vi "Autonomous Independent.vi"   [LabVIEW 2013]
doc: "This VI is called when autonomous begins, and will automatically be terminated when autonomous ends. You can carry out timed or sensor driven robot movement independently without needing to return to the caller."
uses:
  <vilib>/Rock Robotics/WPI/Solenoid/WPI_SolenoidValue.ctl
  Robot Global Data.vi
  <vilib>/Rock Robotics/WPI/RobotDrive/WPI_RobotDriveGetSetRefNum.vi
  <vilib>/Rock Robotics/WPI/Solenoid/WPI_SolenoidSetEnum.vi
  <vilib>/Rock Robotics/WPI/RobotDrive/WPI_RobotDriveArcadeDrive_Standard(NoSaturation).vi
  <vilib>/Rock Robotics/WPI/Solenoid/Deprecated/WPI_SolenoidGetBool.vi
  <vilib>/Rock Robotics/WPI/Joystick/WPI_JoystickGetSetRefNum.vi
panel:
  # "Be sure to right-click and choose Data Operations>>Make Current Value default if you want to save the array values with the VI"
types:
  T1 = typedef "WPI_JoystickDevRef.ctl" = cluster{"Device":T2}
  T2 = typedef "WPI_JoystickDeviceEnum.ctl" = enum16{"USB 1", "USB 2", "USB 3", "USB 4", "Kinect 1", "Kinect 2"}
  T3 = cluster{"axis 1 (x)":dbl, "axis 2 (y)":dbl, "axis 3 (throttle)":dbl, "axis 4":dbl, "axis 5":dbl, "axis 6":dbl}
  T4 = typedef "WPI_MotorControlDeviceRef.ctl" = cluster{"DeviceStatus":errorcluster, "Type":enum16{"PWM", "CAN"}, "PWM":cluster{"Digital Module":T5, "PWM Channel":T6, "DeadBand":T7}, "CAN":cluster{"Device Number":u8, "Control Mode":T8, "Semaphore":T9, "Max Vout":dbl}, "Invert":bool, "TransformRef":T10, "InvTransformRef":T10}
  T5 = typedef "FPGA_TypedefDigitalModule.ctl" = enum16{"Digital Module 1", "Digital Module 2"}
  T6 = typedef "FPGA_DIOPWMChannel.ctl" = enum8{"PWM 1", "PWM 2", "PWM 3", "PWM 4", "PWM 5", "PWM 6", "PWM 7", "PWM 8", "PWM 9", "PWM 10", "Invalid"}
  T7 = typedef "WPI_PWMDeadband.ctl" = cluster{"Name":string, "maxPositivePwm":i32, "minPositivePwm":i32, "centerPwm":i32, "maxNegativePwm":i32, "minNegativePwm":i32, "angularRange":u16}
  T8 = typedef "WPI_CANJaguar_ControlMode.ctl" = enum8{"Percent VBus", "Current", "Speed", "Position", "Voltage"}
  T9 = typedef "Semaphore RefNum" = refnum<k1>
  T10 = typedef "WPI_PWMTransform_ConPane.ctl" = refnum<vi>
  T11 = typedef "WPI_SolenoidDevRef.ctl" = cluster{"DevStatus":errorcluster, "Solenoid Module":T12, "Forward Solenoid Channel":T13, "Reverse Solenoid Channel":T13}
  T12 = typedef "FPGA_TypedefSolenoidModule.ctl" = enum16{"Solenoid Module 1", "Solenoid Module 2"}
  T13 = typedef "WPI_SolenoidChannel.ctl" = enum8{"Solenoid 1", "Solenoid 2", "Solenoid 3", "Solenoid 4", "Solenoid 5", "Solenoid 6", "Solenoid 7", "Solenoid 8", "Invalid"}
  T14 = typedef "WPI_RobotDriveDevRef.ctl" = cluster{"DevStatus":errorcluster, "Motors[]":T4[], "Square Inputs":bool, "Max Output":dbl, "Isochronous":bool}
  T15 = typedef "WPI_SolenoidValue.ctl" = enum16{"Off", "On", "Forward", "Reverse"}
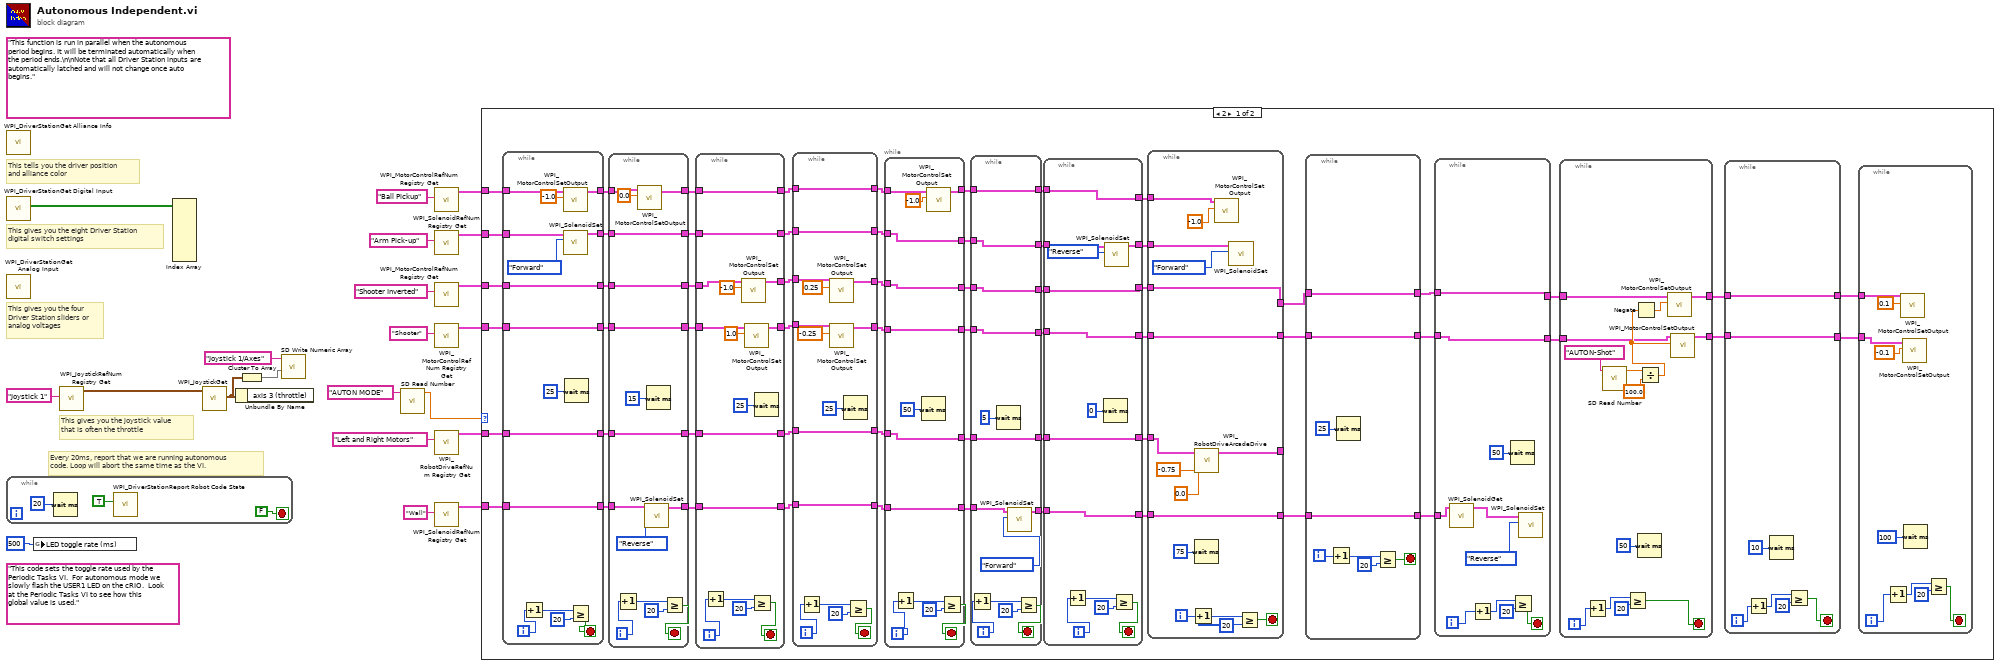
[diagram p0: block diagram]
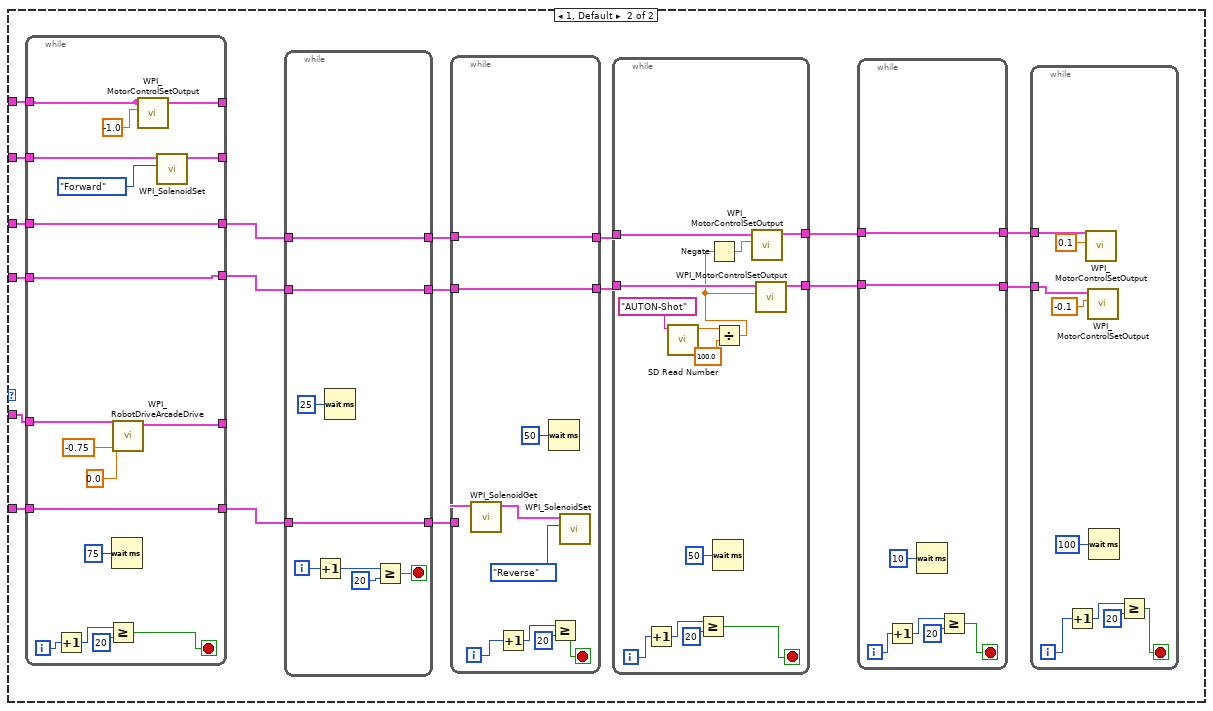
[diagram p2: hidden frame]
diagram:
  (unwired) "This code sets the toggle rate used by the Periodic Tasks VI.  For autonomous mode we slowly flash the USER1 LED on the cRIO.  Look at the Periodic Tasks VI to see how this global value is used."
  (unwired) "This function is run in parallel when the autonomous period begins. It will be terminated automatically when the period ends.\n\nNote that all Driver Station inputs are automatically latched and will not change once auto begins."
  # "Every 20ms, report that we are running autonomous\ncode. Loop will abort the same time as the VI."
  # "This gives you the joystick value\nthat is often the throttle"
  # "This tells you the driver position\nand alliance color"
  # "This gives you the eight Driver Station\ndigital switch settings"
  # "This gives you the four\nDriver Station sliders or\nanalog voltages"
  n1 = call <vilib>:"WPI_DriverStationGet Alliance Info.vi"() -> ()  [unwired: 12 out]
  n2 = call <vilib>:"WPI_DriverStationGet Digital Input.vi"() -> ("Driver Station Digital Input (1-8)"=w21:bool[])  [unwired: 11 out]
  n3 = call <vilib>:"WPI_DriverStationGet Analog Input.vi"() -> ()  [unwired: 12 out]
  n4 = while {
    stop <- FALSE stop-if-true
    n5 = Wait (ms)(milliseconds to wait=u32 20) -> ()  [unwired: 1 out]
    n6 = call <vilib>:"WPI_DriverStationReport Robot Code State.vi"("Autonomous"=TRUE) -> ()  [unwired: 10 in, 1 out]
  }
  n7 = global write "Robot Global Data.vi" "LED toggle rate (ms)"(u32 500 ("LED ms toggle rate")) -> ()
  n8 = call <vilib>:"WPI_JoystickRefNum Registry Get.vi"("refnum name"="Joystick 1") -> ("JoystickDevRef"=w19:T1)  [unwired: 1 in, 9 out]
  n9 = Index Array(array=w21) -> ()  [unwired: 8 in, 8 out]
  n10 = call <vilib>:"WPI_JoystickGet.vi"("JoystickDevRef"=w19) -> ("Axes"=w16:T3)  [unwired: 1 in, 5 out]
  n11 = Unbundle By Name(w16) -> ()  [unwired: 1 out]
  n12 = Cluster To Array(cluster=w16) -> (array=w17:dbl[])
  n13 = call <vilib>:"SD Write Numeric Array.vi"("Numeric Array"=w17, "Name"="Joystick 1/Axes") -> ()  [unwired: 8 in, 2 out]
  n14 = call <vilib>:"SD Read Number.vi"("Name"="AUTON MODE") -> ("Numeric"=w13:dbl)  [unwired: 8 in, 2 out]
  n15 = call <vilib>:"WPI_MotorControlRefNum Registry Get.vi"("refnum name"="Ball Pickup") -> ("MotorControlDevRef"=w1:T4)  [unwired: 9 in, 1 out]
  n16 = call <vilib>:"WPI_SolenoidRefNum Registry Get.vi"("refnum name"="Arm Pick-up") -> ("SolenoidDevRef"=w2:T11)  [unwired: 9 in, 1 out]
  n17 = call <vilib>:"WPI_MotorControlRefNum Registry Get.vi"("refnum name"="Shooter Inverted") -> ("MotorControlDevRef"=w3:T4)  [unwired: 9 in, 1 out]
  n18 = call <vilib>:"WPI_MotorControlRefNum Registry Get.vi"("refnum name"="Shooter") -> ("MotorControlDevRef"=w4:T4)  [unwired: 9 in, 1 out]
  n19 = call <vilib>:"WPI_RobotDriveRefNum Registry Get.vi"("refnum name"="Left and Right Motors") -> ("RobotDriveDevRef"=w6:T14)  [unwired: 9 in, 1 out]
  n20 = call <vilib>:"WPI_SolenoidRefNum Registry Get.vi"("refnum name"="Wall") -> ("SolenoidDevRef"=w5:T11)  [unwired: 9 in, 1 out]
  n21 = case shown="2" w13 {
    tunnel: w6 -> [w76 w265]
    tunnel: w5 -> [w75 w254]
    tunnel: w4 -> [w77 w264]
    tunnel: w3 -> [w78 w263]
    tunnel: w2 -> [w80 w262]
    tunnel: w1 -> [w79 w261]
    frame 2 {
      n22 = while {
        tunnel: w80 -> [w179]
        tunnel: w79 -> [w177]
        tunnel: [w175] -> w71
        tunnel: w78 -> [w175]
        tunnel: w77 -> [w174]
        tunnel: [w174] -> w72
        tunnel: w76 -> [w173]
        tunnel: [w173] -> w73
        tunnel: w75 -> [w172]
        tunnel: [w172] -> w74
        tunnel: [w170] -> w70
        tunnel: [w169] -> w69
        i -> [w180]
        stop <- w181 stop-if-true
        n23 = Increment(x=w180) -> (x+1=w183:i32)
        n24 = call <vilib>:"WPI_MotorControlSetOutput.vi"("Output"=-1.0, "MotorControlDevRef"=w177) -> ("MotorControlDevRef"=w169:T4)  [unwired: 7 in, 2 out]
        n25 = call-poly <vilib>:"WPI_SolenoidSet.vi"("Value"=WPI_SolenoidValue."Forward", "SolenoidDevRef"=w179) -> ("SolenoidDevRef"=w170:T11)  [unwired: 8 in, 1 out]
        n26 = Wait (ms)(milliseconds to wait=u32 25) -> ()  [unwired: 1 out]
        n27 = Greater Or Equal?(x=w183, y=20) -> (x >= y?=w181:bool)
      }
      n28 = while {
        tunnel: w74 -> [w168]
        tunnel: w73 -> [w161]
        tunnel: w72 -> [w160]
        tunnel: w71 -> [w159]
        tunnel: w70 -> [w158]
        tunnel: w69 -> [w156]
        tunnel: [w161] -> w64
        tunnel: [w160] -> w65
        tunnel: [w159] -> w66
        tunnel: [w158] -> w67
        tunnel: [w155] -> w68
        tunnel: [w157] -> w63
        i -> [w163]
        stop <- w164 stop-if-true
        n29 = Increment(x=w163) -> (x+1=w165:i32)
        n30 = call <vilib>:"WPI_MotorControlSetOutput.vi"("Output"=0.0, "MotorControlDevRef"=w156) -> ("MotorControlDevRef"=w155:T4)  [unwired: 7 in, 2 out]
        n31 = call-poly <vilib>:"WPI_SolenoidSet.vi"("Value"=WPI_SolenoidValue."Reverse", "SolenoidDevRef"=w168) -> ("SolenoidDevRef"=w157:T11)  [unwired: 8 in, 1 out]
        n32 = Wait (ms)(milliseconds to wait=u32 15) -> ()  [unwired: 1 out]
        n33 = Greater Or Equal?(x=w165, y=20) -> (x >= y?=w164:bool)
      }
      n34 = while {
        tunnel: w68 -> [w153]
        tunnel: w67 -> [w152]
        tunnel: w66 -> [w150]
        tunnel: w65 -> [w151]
        tunnel: w64 -> [w147]
        tunnel: w63 -> [w146]
        tunnel: [w153] -> w62
        tunnel: [w152] -> w61
        tunnel: [w147] -> w58
        tunnel: [w146] -> w57
        tunnel: [w145] -> w60
        tunnel: [w144] -> w59
        i -> [w140]
        stop <- w141 stop-if-true
        n35 = Increment(x=w140) -> (x+1=w143:i32)
        n36 = call <vilib>:"WPI_MotorControlSetOutput.vi"("Output"=-1.0, "MotorControlDevRef"=w150) -> ("MotorControlDevRef"=w145:T4)  [unwired: 7 in, 2 out]
        n37 = call <vilib>:"WPI_MotorControlSetOutput.vi"("Output"=1.0, "MotorControlDevRef"=w151) -> ("MotorControlDevRef"=w144:T4)  [unwired: 7 in, 2 out]
        n38 = Greater Or Equal?(x=w143, y=20) -> (x >= y?=w141:bool)
        n39 = Wait (ms)(milliseconds to wait=u32 25) -> ()  [unwired: 1 out]
      }
      n40 = while {
        tunnel: w62 -> [w134]
        tunnel: w61 -> [w133]
        tunnel: w60 -> [w137]
        tunnel: w59 -> [w138]
        tunnel: [w134] -> w51
        tunnel: [w133] -> w52
        tunnel: w58 -> [w131]
        tunnel: w57 -> [w132]
        tunnel: [w132] -> w56
        tunnel: [w131] -> w55
        tunnel: [w130] -> w54
        tunnel: [w129] -> w53
        i -> [w125]
        stop <- w126 stop-if-true
        n41 = Increment(x=w125) -> (x+1=w127:i32)
        n42 = call <vilib>:"WPI_MotorControlSetOutput.vi"("Output"=-0.25, "MotorControlDevRef"=w138) -> ("MotorControlDevRef"=w130:T4)  [unwired: 7 in, 2 out]
        n43 = call <vilib>:"WPI_MotorControlSetOutput.vi"("Output"=0.25, "MotorControlDevRef"=w137) -> ("MotorControlDevRef"=w129:T4)  [unwired: 7 in, 2 out]
        n44 = Wait (ms)(milliseconds to wait=u32 25) -> ()  [unwired: 1 out]
        n45 = Greater Or Equal?(x=w127, y=20) -> (x >= y?=w126:bool)
      }
      n46 = while {
        tunnel: w56 -> [w116]
        tunnel: w55 -> [w115]
        tunnel: w54 -> [w114]
        tunnel: w53 -> [w113]
        tunnel: w52 -> [w112]
        tunnel: w51 -> [w123]
        tunnel: [w116] -> w50
        tunnel: [w115] -> w45
        tunnel: [w114] -> w46
        tunnel: [w113] -> w47
        tunnel: [w112] -> w49
        tunnel: [w111] -> w48
        i -> [w118]
        stop <- w119 stop-if-true
        n47 = Increment(x=w118) -> (x+1=w121:i32)
        n48 = Wait (ms)(milliseconds to wait=u32 50) -> ()  [unwired: 1 out]
        n49 = call <vilib>:"WPI_MotorControlSetOutput.vi"("Output"=-1.0, "MotorControlDevRef"=w123) -> ("MotorControlDevRef"=w111:T4)  [unwired: 7 in, 2 out]
        n50 = Greater Or Equal?(x=w121, y=20) -> (x >= y?=w119:bool)
      }
      n51 = while {
        tunnel: w50 -> [w104]
        tunnel: w49 -> [w99]
        tunnel: w48 -> [w98]
        tunnel: w47 -> [w100]
        tunnel: w46 -> [w101]
        tunnel: w45 -> [w102]
        tunnel: [w103] -> w36
        tunnel: [w102] -> w44
        tunnel: [w101] -> w42
        tunnel: [w100] -> w41
        tunnel: [w99] -> w40
        tunnel: [w98] -> w37
        i -> [w107]
        stop <- w106 stop-if-true
        n52 = Increment(x=w107) -> (x+1=w108:i32)
        n53 = Wait (ms)(milliseconds to wait=u32 5) -> ()  [unwired: 1 out]
        n54 = call-poly <vilib>:"WPI_SolenoidSet.vi"("Value"=WPI_SolenoidValue."Forward", "SolenoidDevRef"=w104) -> ("SolenoidDevRef"=w103:T11)  [unwired: 8 in, 1 out]
        n55 = Greater Or Equal?(x=w108, y=20) -> (x >= y?=w106:bool)
      }
      n56 = while {
        tunnel: [w97] -> w43
        tunnel: w44 -> [w97]
        tunnel: w42 -> [w96]
        tunnel: [w96] -> w29
        tunnel: [w95] -> w28
        tunnel: w41 -> [w95]
        tunnel: w40 -> [w88]
        tunnel: [w87] -> w39
        tunnel: [w94] -> w38
        tunnel: w37 -> [w94]
        tunnel: [w93] -> w35
        tunnel: w36 -> [w93]
        i -> [w89]
        stop <- w90 stop-if-true
        n57 = Increment(x=w89) -> (x+1=w92:i32)
        n58 = Wait (ms)(milliseconds to wait=u32 0) -> ()  [unwired: 1 out]
        n59 = call-poly <vilib>:"WPI_SolenoidSet.vi"("Value"=WPI_SolenoidValue."Reverse", "SolenoidDevRef"=w88) -> ("SolenoidDevRef"=w87:T11)  [unwired: 8 in, 1 out]
        n60 = Greater Or Equal?(x=w92, y=20) -> (x >= y?=w90:bool)
      }
      n61 = while {
        tunnel: [w242] -> _
        tunnel: w43 -> [w237]
        tunnel: w39 -> [w236]
        tunnel: w38 -> [w235]
        tunnel: [w234] -> w33
        tunnel: w35 -> [w234]
        tunnel: [w233] -> w30
        tunnel: w29 -> [w233]
        tunnel: w28 -> [w232]
        tunnel: [w232] -> w27
        i -> [w247]
        stop <- w244 stop-if-true
        n62 = Increment(x=w247) -> (x+1=w246:i32)
        n63 = Wait (ms)(milliseconds to wait=u32 75) -> ()  [unwired: 1 out]
        n64 = call-poly <vilib>:"WPI_RobotDriveArcadeDrive.vi"("Y axis value"=-0.75, "X axis value"=0.0, "RobotDriveDevRef"=w237) -> ("RobotDriveDevRef"=w242:T14)  [unwired: 6 in, 2 out]
        n65 = call <vilib>:"WPI_MotorControlSetOutput.vi"("Output"=-1.0, "MotorControlDevRef"=w235) -> ()  [unwired: 7 in, 3 out]
        n66 = call-poly <vilib>:"WPI_SolenoidSet.vi"("Value"=WPI_SolenoidValue."Forward", "SolenoidDevRef"=w236) -> ()  [unwired: 8 in, 2 out]
        n67 = Greater Or Equal?(x=w246, y=20) -> (x >= y?=w244:bool)
      }
      n68 = while {
        tunnel: [w186] -> w34
        tunnel: w33 -> [w186]
        tunnel: [w185] -> w31
        tunnel: w30 -> [w185]
        tunnel: w27 -> [w184]
        tunnel: [w184] -> w26
        i -> [w189]
        stop <- w188 stop-if-true
        n69 = Increment(x=w189) -> (x+1=w190:i32)
        n70 = Wait (ms)(milliseconds to wait=u32 25) -> ()  [unwired: 1 out]
        n71 = Greater Or Equal?(x=w190, y=20) -> (x >= y?=w188:bool)
      }
      n72 = while {
        tunnel: w34 -> [w224]
        tunnel: [w223] -> w32
        tunnel: w31 -> [w223]
        tunnel: w26 -> [w222]
        tunnel: [w222] -> w25
        i -> [w229]
        stop <- w228 stop-if-true
        n73 = call-poly <vilib>:"WPI_SolenoidGet.vi"("SolenoidDevRef"=w224) -> ("SolenoidDevRef"=w225:T11)  [unwired: 8 in, 2 out]
        n74 = Increment(x=w229) -> (x+1=w230:i32)
        n75 = Wait (ms)(milliseconds to wait=u32 50) -> ()  [unwired: 1 out]
        n76 = Greater Or Equal?(x=w230, y=20) -> (x >= y?=w228:bool)
        n77 = call-poly <vilib>:"WPI_SolenoidSet.vi"("Value"=WPI_SolenoidValue."Reverse", "SolenoidDevRef"=w225) -> ()  [unwired: 8 in, 2 out]
      }
      n78 = while {
        tunnel: [w217] -> w84
        tunnel: [w216] -> w83
        tunnel: w32 -> [w209]
        tunnel: w25 -> [w208]
        i -> [w219]
        stop <- w218 stop-if-true
        n79 = Increment(x=w219) -> (x+1=w221:i32)
        n80 = call <vilib>:"SD Read Number.vi"("Name"="AUTON-Shot") -> ("Numeric"=w212:dbl)  [unwired: 8 in, 2 out]
        n81 = Greater Or Equal?(x=w221, y=20) -> (x >= y?=w218:bool)
        n82 = Wait (ms)(milliseconds to wait=u32 50) -> ()  [unwired: 1 out]
        n83 = Divide(x=w212, y=100.0) -> (x/y=w211:dbl)
        n84 = Negate(x=w211) -> (-x=w213:dbl)
        n85 = call <vilib>:"WPI_MotorControlSetOutput.vi"("Output"=w213, "MotorControlDevRef"=w208) -> ("MotorControlDevRef"=w216:T4)  [unwired: 7 in, 2 out]
        n86 = call <vilib>:"WPI_MotorControlSetOutput.vi"("Output"=w211, "MotorControlDevRef"=w209) -> ("MotorControlDevRef"=w217:T4)  [unwired: 7 in, 2 out]
      }
      n87 = while {
        tunnel: w84 -> [w203]
        tunnel: w83 -> [w202]
        tunnel: [w203] -> w81
        tunnel: [w202] -> w82
        i -> [w204]
        stop <- w205 stop-if-true
        n88 = Increment(x=w204) -> (x+1=w206:i32)
        n89 = Wait (ms)(milliseconds to wait=u32 10) -> ()  [unwired: 1 out]
        n90 = Greater Or Equal?(x=w206, y=20) -> (x >= y?=w205:bool)
      }
      n91 = while {
        tunnel: w82 -> [w199]
        tunnel: w81 -> [w200]
        i -> [w194]
        stop <- w193 stop-if-true
        n92 = Increment(x=w194) -> (x+1=w196:i32)
        n93 = call <vilib>:"WPI_MotorControlSetOutput.vi"("Output"=0.1, "MotorControlDevRef"=w199) -> ()  [unwired: 7 in, 3 out]
        n94 = call <vilib>:"WPI_MotorControlSetOutput.vi"("Output"=-0.1, "MotorControlDevRef"=w200) -> ()  [unwired: 7 in, 3 out]
        n95 = Wait (ms)(milliseconds to wait=u32 100) -> ()  [unwired: 1 out]
        n96 = Greater Or Equal?(x=w196, y=20) -> (x >= y?=w193:bool)
      }
    }
    frame 1, Default {
      n97 = while {
        tunnel: w265 -> [w325]
        tunnel: [w323] -> _
        tunnel: [w322] -> w251
        tunnel: w264 -> [w322]
        tunnel: w263 -> [w321]
        tunnel: [w321] -> w248
        tunnel: w262 -> [w316]
        tunnel: w261 -> [w315]
        tunnel: [w315] -> _
        tunnel: [w316] -> _
        tunnel: [w318] -> w253
        tunnel: w254 -> [w318]
        i -> [w329]
        stop <- w326 stop-if-true
        n98 = Increment(x=w329) -> (x+1=w328:i32)
        n99 = Greater Or Equal?(x=w328, y=20) -> (x >= y?=w326:bool)
        n100 = Wait (ms)(milliseconds to wait=u32 75) -> ()  [unwired: 1 out]
        n101 = call-poly <vilib>:"WPI_RobotDriveArcadeDrive.vi"("Y axis value"=-0.75, "X axis value"=0.0, "RobotDriveDevRef"=w325) -> ("RobotDriveDevRef"=w323:T14)  [unwired: 6 in, 2 out]
        n102 = call <vilib>:"WPI_MotorControlSetOutput.vi"("Output"=-1.0, "MotorControlDevRef"=w315) -> ()  [unwired: 7 in, 3 out]
        n103 = call-poly <vilib>:"WPI_SolenoidSet.vi"("Value"=WPI_SolenoidValue."Forward", "SolenoidDevRef"=w316) -> ()  [unwired: 8 in, 2 out]
      }
      n104 = while {
        tunnel: w253 -> [w273]
        tunnel: [w273] -> w252
        tunnel: w251 -> [w272]
        tunnel: [w272] -> w250
        tunnel: [w271] -> w249
        tunnel: w248 -> [w271]
        i -> [w268]
        stop <- w267 stop-if-true
        n105 = Increment(x=w268) -> (x+1=w269:i32)
        n106 = Wait (ms)(milliseconds to wait=u32 25) -> ()  [unwired: 1 out]
        n107 = Greater Or Equal?(x=w269, y=20) -> (x >= y?=w267:bool)
      }
      n108 = while {
        tunnel: w250 -> [w308]
        tunnel: w249 -> [w309]
        tunnel: [w309] -> w260
        tunnel: [w308] -> w259
        tunnel: w252 -> [w306]
        i -> [w311]
        stop <- w310 stop-if-true
        n109 = call-poly <vilib>:"WPI_SolenoidGet.vi"("SolenoidDevRef"=w306) -> ("SolenoidDevRef"=w304:T11)  [unwired: 8 in, 2 out]
        n110 = Increment(x=w311) -> (x+1=w312:i32)
        n111 = Wait (ms)(milliseconds to wait=u32 50) -> ()  [unwired: 1 out]
        n112 = Greater Or Equal?(x=w312, y=20) -> (x >= y?=w310:bool)
        n113 = call-poly <vilib>:"WPI_SolenoidSet.vi"("Value"=WPI_SolenoidValue."Reverse", "SolenoidDevRef"=w304) -> ()  [unwired: 8 in, 2 out]
      }
      n114 = while {
        tunnel: w260 -> [w299]
        tunnel: w259 -> [w298]
        tunnel: [w297] -> w258
        tunnel: [w296] -> w257
        i -> [w301]
        stop <- w300 stop-if-true
        n115 = Increment(x=w301) -> (x+1=w303:i32)
        n116 = call <vilib>:"SD Read Number.vi"("Name"="AUTON-Shot") -> ("Numeric"=w292:dbl)  [unwired: 8 in, 2 out]
        n117 = Greater Or Equal?(x=w303, y=20) -> (x >= y?=w300:bool)
        n118 = Wait (ms)(milliseconds to wait=u32 50) -> ()  [unwired: 1 out]
        n119 = Divide(x=w292, y=100.0) -> (x/y=w291:dbl)
        n120 = Negate(x=w291) -> (-x=w293:dbl)
        n121 = call <vilib>:"WPI_MotorControlSetOutput.vi"("Output"=w293, "MotorControlDevRef"=w299) -> ("MotorControlDevRef"=w296:T4)  [unwired: 7 in, 2 out]
        n122 = call <vilib>:"WPI_MotorControlSetOutput.vi"("Output"=w291, "MotorControlDevRef"=w298) -> ("MotorControlDevRef"=w297:T4)  [unwired: 7 in, 2 out]
      }
      n123 = while {
        tunnel: w258 -> [w285]
        tunnel: w257 -> [w284]
        tunnel: [w285] -> w255
        tunnel: [w284] -> w256
        i -> [w286]
        stop <- w287 stop-if-true
        n124 = Increment(x=w286) -> (x+1=w288:i32)
        n125 = Wait (ms)(milliseconds to wait=u32 10) -> ()  [unwired: 1 out]
        n126 = Greater Or Equal?(x=w288, y=20) -> (x >= y?=w287:bool)
      }
      n127 = while {
        tunnel: w256 -> [w281]
        tunnel: w255 -> [w282]
        i -> [w276]
        stop <- w275 stop-if-true
        n128 = Increment(x=w276) -> (x+1=w278:i32)
        n129 = call <vilib>:"WPI_MotorControlSetOutput.vi"("Output"=0.1, "MotorControlDevRef"=w281) -> ()  [unwired: 7 in, 3 out]
        n130 = call <vilib>:"WPI_MotorControlSetOutput.vi"("Output"=-0.1, "MotorControlDevRef"=w282) -> ()  [unwired: 7 in, 3 out]
        n131 = Wait (ms)(milliseconds to wait=u32 100) -> ()  [unwired: 1 out]
        n132 = Greater Or Equal?(x=w278, y=20) -> (x >= y?=w275:bool)
      }
    }
  }
